vi "Verify GPS Data.vi"(1 "GPS Point":T1 {"Longitude" format="%#_14g"; "Latitude" format="%#_14g"}) -> (0 "Data OK?":bool)   [LabVIEW 2009]
uses:
  TypeDefs/Sensor Typedefs/GPS Data.ctl
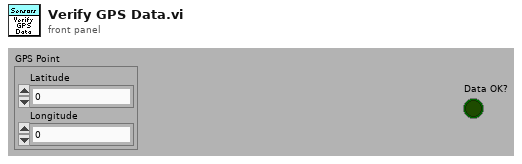
[diagram p1: front panel]
types:
  T1 = typedef "GPS Data.ctl" = cluster{"Latitude":dbl, "Longitude":dbl}
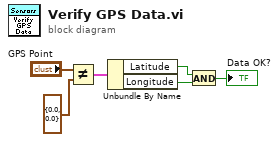
[diagram p0: block diagram]
diagram:
  n1 = Not Equal?(x="GPS Point", y=T1 {"Latitude"=0.0, "Longitude"=0.0} ("GPS Point")) -> (x != y?=w4:cluster{"Latitude":bool, "Longitude":bool})
  n2 = Unbundle By Name(w4) -> ("Latitude"=w3:bool, "Longitude"=w2:bool)
  n3 = And(x=w3, y=w2) -> (x .and. y?=→"Data OK?":bool)
